vi "2D Complex FFT.vi"(8 "n":i32=-1, 9 "m":i32=-1, 10 "shift?":bool, 11 "X":cdb[][](array[numeric])) -> (0 "error":i32, 3 "FFT {X}":cdb[][](array[numeric]))   [LabVIEW 2017, in "NI_AALPro.lvlib"]
doc: "Computes the fast Fourier transform (FFT) of the input sequence <B>X</B>. Wire data to the <B>X</B> input to determine the polymorphic instance to use or manually select the instance."
uses:
  <vilib>/Analysis/NI_AALPro.lvlib
  <resource>/lvanlys.dll
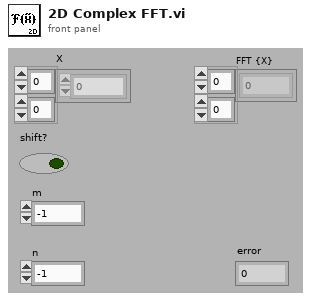
[diagram p1: front panel]
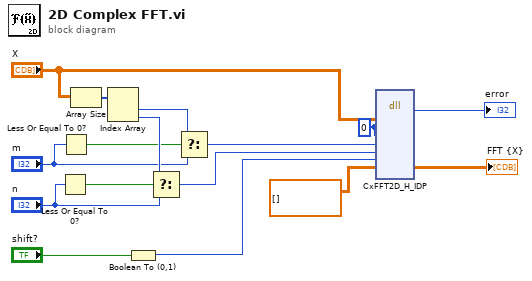
[diagram p0: block diagram]
diagram:
  w1 = 0 ("orgRow")
  n1 = Less Or Equal To 0?(x="n") -> (x <= 0?=w8:bool)
  n2 = Less Or Equal To 0?(x="m") -> (x <= 0?=w9:bool)
  n3 = Array Size(array="X") -> (size(s)=w15:i32[])
  n4 = Index Array(array=w15) -> (element #1=w14:i32, element #2=w13:i32)  [unwired: 2 in]
  n5 = Boolean To (0,1)(Boolean="shift?") -> (0, 1=w5:i16)
  n6 = Select(t=w13, s=w8, f="n") -> (s? t:f=w11:i32)
  n7 = Select(t=w14, s=w9, f="m") -> (s? t:f=w12:i32)
  n8 = dll-call lib="e:/builds/penguin/labview/branches/2017/dev/dist/resource/lvanlys.*" fn="CxFFT2D_H_IDP"("xH"="X", "orgRow"=w1, "orgCol"=w1, "rowsFFT"=w12, "colsFFT"=w11, "shift"=w5, "yH"=cdb[][] [] ("FFT {X}")) -> ("return type"=→"error":i32, "yH"=→"FFT {X}":cdb[][])  [unwired: 11 in, 2 out]
